vi "uTransport_Destroy.vi"(8 "error in (no error)":errorcluster, 11 "uTransport in":refnum<class "uTransport.lvclass">) -> (0 "error out":errorcluster)   [LabVIEW 2021, in "uFramework.lvlib" / "uTransport.lvclass"]
uses:
  uTransport.lvclass
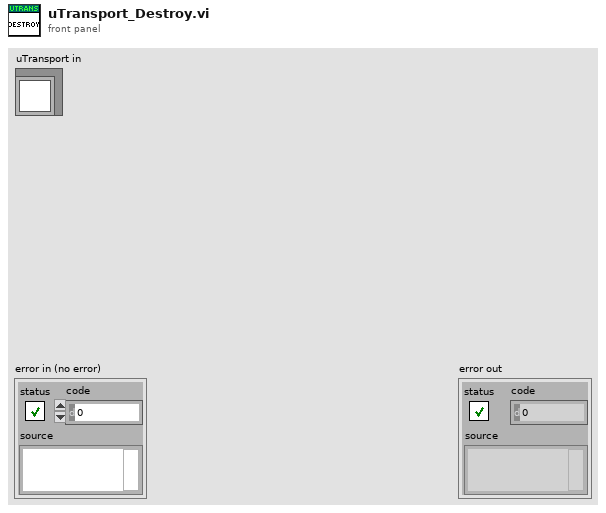
[diagram p1: front panel]
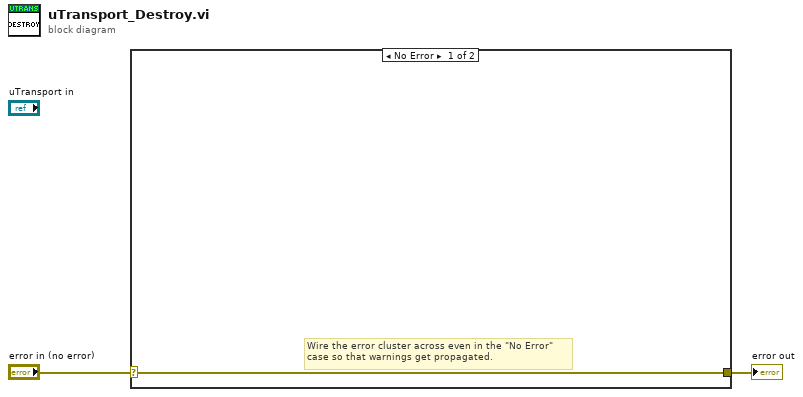
[diagram p0: block diagram]
diagram:
  n1 = case shown="No Error" "error in (no error)" {
    selector: "error in (no error)" -> [w3 w4]
    tunnel: [w3 w4] -> w1
    frame No Error {
      # "Wire the error cluster across even in the \"No Error\"\ncase so that warnings get propagated."
    }
    frame Error {
    }
  }
  "error out" <- w1
